vi "CC Observation Check For BlockID.vi"(8 "error in (no error)":errorcluster, 9 "Generate ID?":bool, 10 "BlockID":string, 11 "Observation List":T1[](array[typedef])) -> (0 "error out":errorcluster, 2 "BlockID string":string, 3 "Found?":bool)   [LabVIEW 2024]
uses:
  typedefs/CC cluster Observation.ctl
  CC enum Observation Status.ctl
  Telescope/CC cluster Telescope Offsets.ctl
  typedefs/CC cluster Observation Dither Options.ctl
  typedefs/CC enum Dither Selection.ctl
  typedefs/CC cluster RA and DEC.ctl
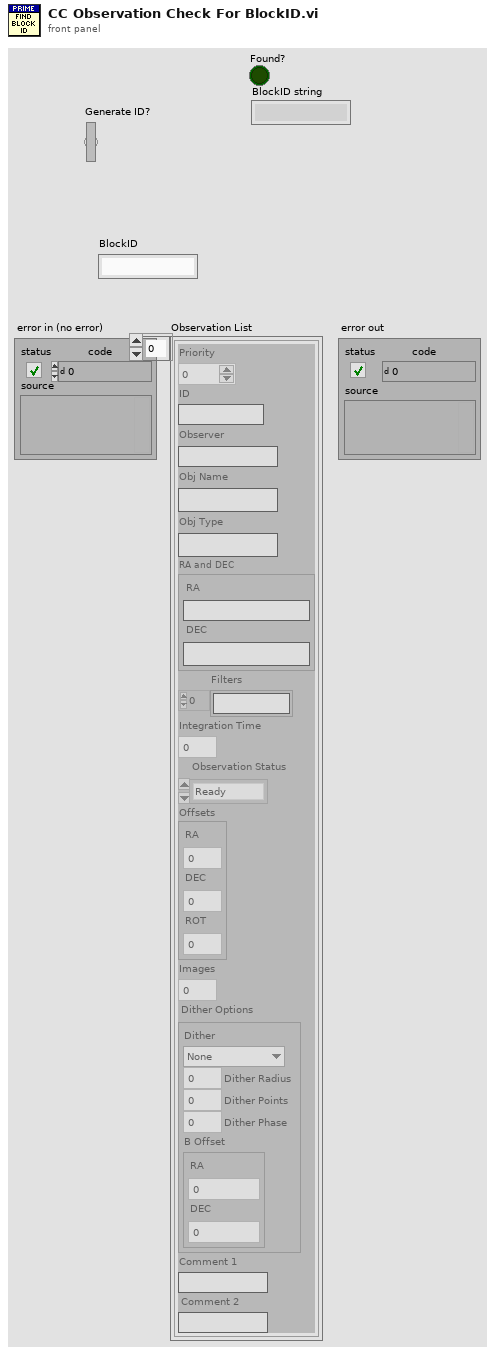
[diagram p1: front panel]
types:
  T1 = typedef "CC cluster Observation.ctl" = cluster{"Priority":i32, "ID":string, "Observer":string, "Obj Name":string, "Obj Type":string, "RA and DEC String":cluster{"RA":string, "DEC":string}, "Filters":string[], "Integration Time":dbl, "Observation Status":T2, "Offsets":T3, "Images":i32, "Dither Options":T4, "Comment 1":string, "Comment 2":string}
  T2 = typedef "CC enum Observation Status.ctl" = enum16{"Ready", "Running", "Done", "Error"}
  T3 = typedef "CC cluster Telescope Offsets.ctl" = cluster{"RA":dbl, "DEC":dbl, "ROT":dbl}
  T4 = typedef "CC cluster Observation Dither Options.ctl" = cluster{"Dither":T5, "Dither Radius":dbl, "Dither Points":i32, "Dither Phase":dbl, "B Offset":T6}
  T5 = typedef "CC enum Dither Selection.ctl" = enum16{"None", "Circle", "Random", "ABBA"}
  T6 = typedef "CC cluster RA and DEC.ctl" = cluster{"RA":dbl, "DEC":dbl}
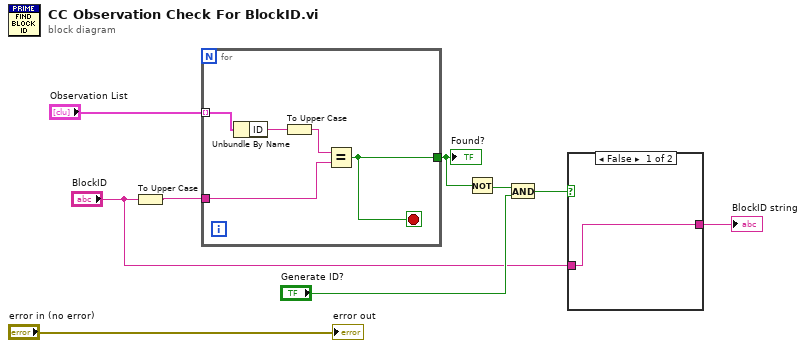
[diagram p0: block diagram]
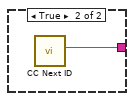
[diagram p2: hidden frame]
diagram:
  n1 = To Upper Case(1:"BlockID") -> (0:w7:string)
  n2 = for {
    tunnel: "Observation List" -> [w14] mode=indexing
    tunnel: w7 -> [w11]
    tunnel: [w10] -> w6
    stop <- w10 stop-if-true
    n3 = Unbundle By Name(w14) -> ("ID"=w13:string)
    n4 = To Upper Case(1:w13) -> (0:w12:string)
    n5 = Equal?(x=w12, y=w11) -> (x = y?=w10:bool)
  }
  "Found?" <- w6
  n6 = Not(x=w6) -> (.not. x?=w5:bool)
  n7 = And(x=w5, y="Generate ID?") -> (x .and. y?=w3:bool)
  n8 = case shown="False" w3 {
    tunnel: [w15 w16] -> w2
    tunnel: "BlockID" -> [w15 _]
    frame False {
    }
    frame True {
      n9 = call "CC Next ID.vi"() -> ("BlockID string"=w16:string)  [unwired: 9 in, 2 out]
    }
  }
  "BlockID string" <- w2
  "error out" <- "error in (no error)"
